vi "Convert Image to RGB565 header file.vi"(8 "error in (no error)":errorcluster, 10 "folder to output file":path, 11 "path to image file (png, jpeg, jpg, bmp)":path) -> (0 "error out":errorcluster)   [LabVIEW 2019, in "LabVIEW RGB565 Convertor.lvlib"]
uses:
  LabVIEW RGB565 Convertor.lvlib
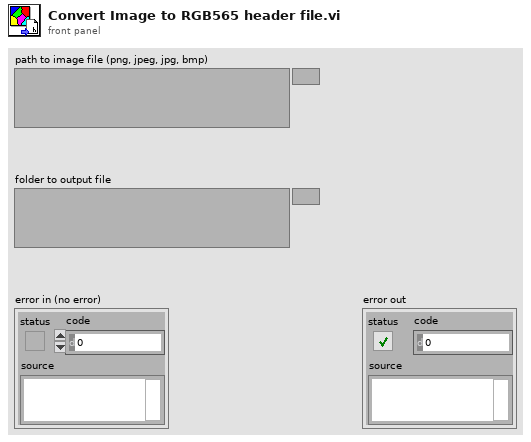
[diagram p1: front panel]
types:
  T1 = typedef "imagedata.ctl" = cluster{"image type":i32, "image depth":i32, "image":u8[], "mask":u8[], "colors":u32[], "Rectangle":cluster{"left":i16, "top":i16, "right":i16, "bottom":i16}}
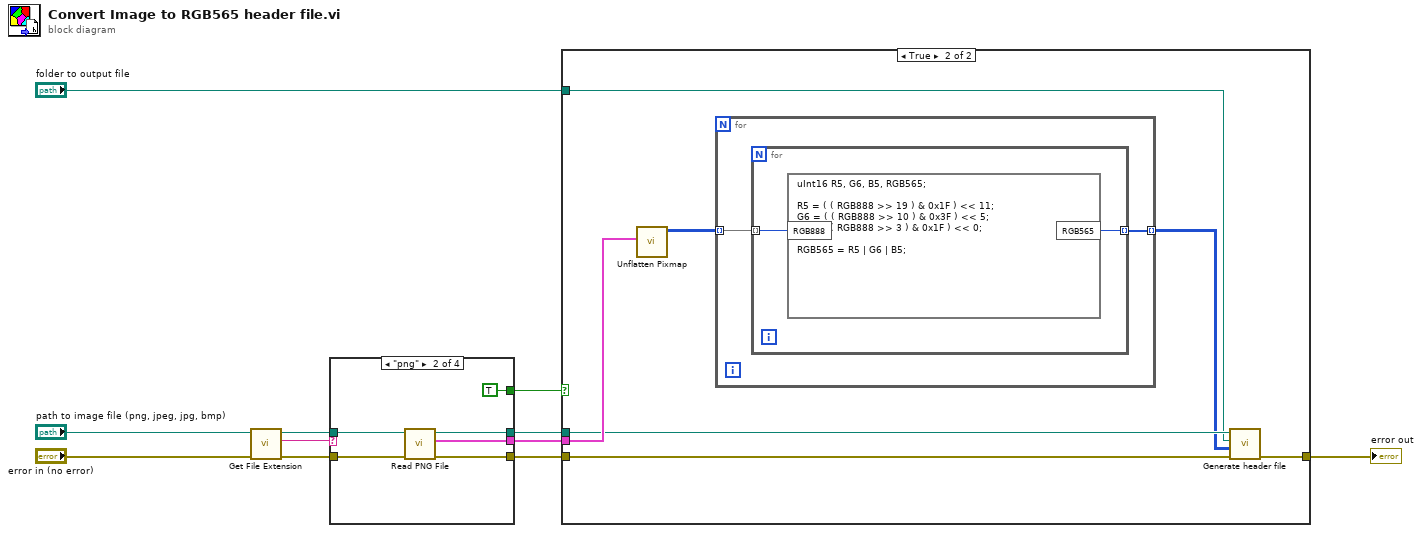
[diagram p0: block diagram]
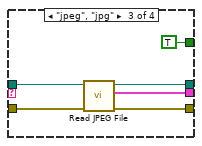
[diagram p4: hidden frame]
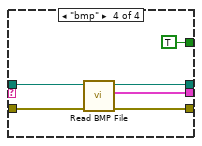
[diagram p5: hidden frame]
diagram:
  n1 = call <vilib>:"Get File Extension.vi"("error in (no error)"="error in (no error)", "file"="path to image file (png, jpeg, jpg, bmp)") -> ("error out"=w8:errorcluster, "lowercase file extension"=w10:string, "dup file"=w5:path)  [unwired: 5 in, 2 out]
  n2 = case shown="\"png\"" w10 {
    tunnel: w5 -> [w12 w19 w25 w31]
    tunnel: [_ w18 w24 w30] -> w9
    tunnel: w8 -> [w13 w17 w23 w29]
    tunnel: [w13 w16 w22 w28] -> w4
    tunnel: [_ TRUE TRUE TRUE] -> w6
    tunnel: [w12 w14 w20 w26] -> w3
    frame Default {
    }
    frame "png" {
      n3 = call <vilib>:"Read PNG File.vi"("error in (no error)"=w17, "path to PNG file"=w19) -> ("error out"=w16:errorcluster, "image data"=w18:T1, "path"=w14:path)  [unwired: 7 in]
    }
    frame "jpeg", "jpg" {
      n4 = call <vilib>:"Read JPEG File.vi"("error in (no error)"=w23, "path to JPEG file"=w25) -> ("error out"=w22:errorcluster, "image data"=w24:T1, "path"=w20:path)  [unwired: 7 in]
    }
    frame "bmp" {
      n5 = call <vilib>:"Read BMP File.vi"("error in (no error)"=w29, "path to BMP file"=w31) -> ("error out"=w28:errorcluster, "image data"=w30:T1, "path"=w26:path)  [unwired: 7 in]
    }
  }
  n6 = case shown="True" w6 {
    tunnel: w9 -> [_ w39]
    tunnel: w4 -> [w32 w36]
    tunnel: w3 -> [_ w37]
    tunnel: "folder to output file" -> [_ w34]
    tunnel: [w32 w33] -> w1
    frame False {
    }
    frame True {
      n7 = call <vilib>:"Unflatten Pixmap.vi"("image data"=w39) -> ("24-bit pixmap"=w38:u32[][])  [unwired: 4 in, 6 out]
      n8 = for {
        tunnel: w38 -> [w41] mode=indexing
        tunnel: [w40] -> w35 mode=indexing
        n9 = for {
          tunnel: w41 -> [w43] mode=indexing
          tunnel: [w42] -> w40 mode=indexing
          n10 = formula code="uInt16 R5, G6, B5, RGB565;\n\nR5 = ( ( RGB888 >> 19 ) & 0x1F ) << 11;\nG6 = ( ( RGB888 >> 10 ) & 0x3F ) << 5;\nB5 = ( ( RGB888 >> 3 ) & 0x1F ) << 0;\n\nRGB565 = R5 | G6 | B5;"("RGB888"=w43) -> ("RGB565"=w42:u16)
        }
      }
      n11 = call "Generate header file.vi"("error in (no error)"=w36, "Pixmap"=w35, "folder to output file"=w34, "path to image file (png, jpeg, jpg, bmp)"=w37) -> ("error out"=w33:errorcluster)  [unwired: 7 in]
    }
  }
  "error out" <- w1
